vi "PH_AWG-510.set Status.vi"(0 "i ref in":refnum<vi>, 5 "error in":errorcluster) -> (14 "i ref out":refnum<vi>, 19 "error out":errorcluster)   [LabVIEW 2014, in "PH_AWG-510.lvlib"]
doc: "This VI sets the status: In case of a device failure it is set to failure (3), otherwise to on (2). The status is indicated and published a DIM-service."
uses:
  PH_AWG-510.lvlib
  PH_Basics/PH_StatusHandler/PH_StatusHandler.Status.ctl
  PH_Basics/PH_StatusHandler/PH_StatusHandler.lvlib
  instr.lib/awg510/Tektronix AWG510.lvlib
  PH_Basics/PH_Common/PH_Common.lvlib
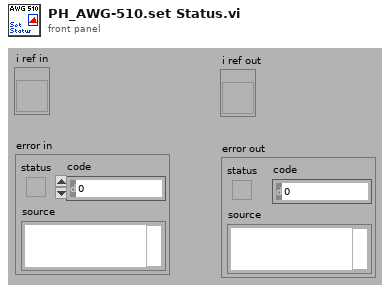
[diagram p1: front panel]
types:
  T1 = typedef "PH_AWG-510.lvlib/PH_AWG-510.i attribute.ctl" = cluster{"GUI Refs":cluster{"Delete":refnum<vi>, "Trigger Settings":refnum<vi>, "Start Device":refnum<vi>, "Instrument Information":refnum<vi>, "Lock Frontpanel":refnum<vi>, "Waveform Pattern File":refnum<vi>, "Initialize":refnum<vi>, "Output Settings":refnum<vi>}, "Instrument Information":T2, "Initialized?":bool, "Current Settings":cluster{"Trigger":T3, "Output Settings":T4}, "Wanted Settings":cluster{"Trigger":T3, "Output Settings":T4}, "Device frontpanel locked?":bool, "Default File Path":path}
  T2 = typedef "PH_AWG-510.lvlib/PH_AWG-510.Instrument Information Dataset.ctl" = cluster{"VISA resource name":refnum<visa-resource-name>, "Instrument Firmware Revision":string, "Manufacturer":string, "Model":string, "Serial Number":string, "Error Message":string, "Device Status":enum16{"stopped", "wating for trigger", "running", "Failure"}}
  T3 = typedef "PH_AWG-510.lvlib/PH_AWG-510.Trigger Settings.ctl" = cluster{"Mode":enum16{"Continuous", "Triggered", "Gated", "Enhanced"}, "Level (V)":dbl, "External Source":bool}
  T4 = typedef "PH_AWG-510.lvlib/PH_AWG-510.Output Settings.ctl" = cluster{"Activate Channel":bool, "VPP (V)":dbl, "Clock (Hz)":dbl, "File Name (Device)":string, "#1":u16, "#2":u16, "#3":u16, "#4":u16, "#5":u16, "#6":u16, "#7":u16, "#8":u16, "#9":u16, "#10":u16, "#11":u16, "#12":u16, "#13":u16, "#14":u16, "#15":u16, "#16":u16, "#17":u16, "#18":u16, "#19":u16, "#20":u16, "Offset (V)":dbl}
  T5 = typedef "PH_StatusHandler.lvlib/PH_StatusHandler.Status.ctl" = i16
  T6 = enum16{"stopped", "wating for trigger", "running"}
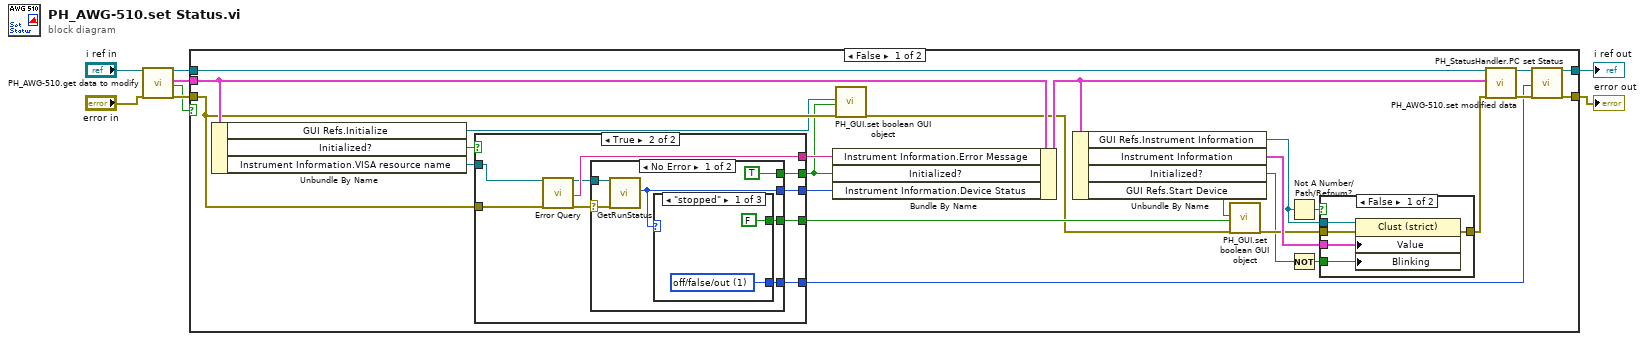
[diagram p0: block diagram]
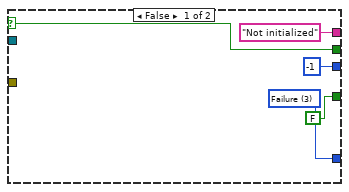
[diagram p2: hidden frame]
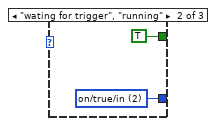
[diagram p3: hidden frame]
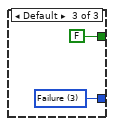
[diagram p4: hidden frame]
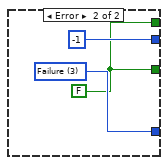
[diagram p5: hidden frame]
diagram:
  n1 = call "PH_AWG-510.get data to modify.vi"("i ref in"="i ref in", "error in (no error)"="error in") -> ("i ref out"=w7:refnum<vi>, "i attribute"=w3:T1, "timed out"=w1:bool, "error out"=w5:errorcluster)  [unwired: 14 in]
  n2 = case shown="False" w1 {
    tunnel: w7 -> [w33 w70]
    tunnel: w5 -> [w20 w69]
    tunnel: [w11 w70] -> w4
    tunnel: w3 -> [w32 _]
    tunnel: [w13 w69] -> w2
    frame False {
      n3 = Unbundle By Name(w32) -> ("GUI Refs.Initialize"=w14:refnum<vi>, "Initialized?"=w28:bool, "Instrument Information.VISA resource name"=w29:refnum<visa-resource-name>)
      n4 = case shown="True" w28 {
        selector: w28 -> [w36 _]
        tunnel: [w37 w47] -> w10
        tunnel: ["Not initialized" ("Error Message") w46] -> w17
        tunnel: w29 -> [_ w45]
        tunnel: w20 -> [_ w44]
        tunnel: [w36 w39] -> w15
        tunnel: [-1 w43] -> w24
        tunnel: [FALSE w42] -> w22
        frame False {
          w37 = T5 3 items=["no info", "off/false/out", "on/true/in", "Failure", "Alarm", "Status 1", "Status 2", "Status 3"] ("f")
        }
        frame True {
          n5 = call "Error Query.vi"("VISA resource name"=w45, "error in (no error)"=w44) -> ("VISA resource name out"=w41:refnum<visa-resource-name>, "Error Message"=w46:string, "error out"=w40:errorcluster)  [unwired: 14 in, 1 out]
          n6 = case shown="No Error" w40 {
            selector: w40 -> [w52 _]
            tunnel: w41 -> [w53 _]
            tunnel: [w51 -1] -> w43
            tunnel: [w50 w61] -> w47
            tunnel: [w49 w60] -> w42
            tunnel: [TRUE w60] -> w39
            frame No Error {
              n7 = call "GetRunStatus.vi"("VISA resource name"=w53, "error in"=w52) -> ("Status"=w51:T6)  [unwired: 15 in, 2 out]
              n8 = case shown="\"stopped\"" w51 {
                tunnel: [w55 w57 w59] -> w50
                tunnel: [FALSE TRUE FALSE] -> w49
                frame "stopped" {
                  w55 = T5 1 items=["no info", "off/false/out", "on/true/in", "Failure", "Alarm", "Status 1", "Status 2", "Status 3"] ("Status")
                }
                frame "wating for trigger", "running" {
                  w57 = T5 2 items=["no info", "off/false/out", "on/true/in", "Failure", "Alarm", "Status 1", "Status 2", "Status 3"] ("Status")
                }
                frame Default {
                  w59 = T5 3 items=["no info", "off/false/out", "on/true/in", "Failure", "Alarm", "Status 1", "Status 2", "Status 3"] ("Status")
                }
              }
            }
            frame Error {
              w60 = FALSE
              w61 = T5 3 items=["no info", "off/false/out", "on/true/in", "Failure", "Alarm", "Status 1", "Status 2", "Status 3"] ("Status")
            }
          }
        }
      }
      n9 = Bundle By Name(cluster=w32, "Instrument Information.Error Message"=w17, "Initialized?"=w15, "Instrument Information.Device Status"=w24) -> (w27:T1)
      n10 = call "PH_GUI.set boolean GUI object.vi"("Boolean Knob GUI Ref"=w14, "Value"=w15, "error in (no error)"=w20) -> ("error out"=w16:errorcluster)  [unwired: 16 in]
      n11 = Unbundle By Name(w27) -> ("GUI Refs.Instrument Information"=w25:refnum<vi>, "Instrument Information"=w26:T2, "Initialized?"=w19:bool, "GUI Refs.Start Device"=w21:refnum<vi>)
      n12 = call "PH_GUI.set boolean GUI object.vi"("Boolean Knob GUI Ref"=w21, "Value"=w22, "error in (no error)"=w16) -> ("error out"=w23:errorcluster)  [unwired: 16 in]
      n13 = Not A Number/Path/Refnum?(number/path/refnum=w25) -> (NaN/Path/Refnum?=w30:bool)
      n14 = Not(x=w19) -> (.not. x?=w18:bool)
      n15 = case shown="False" w30 {
        tunnel: w23 -> [w67 w68]
        tunnel: [w66 w68] -> w9
        tunnel: w25 -> [w65 _]
        tunnel: w18 -> [w63 _]
        tunnel: w26 -> [w64 _]
        frame False {
          n16 = property class="Clust (strict)"(reference=w65, error in=w67, "Value"=w64, "Blinking"=w63) -> (error out=w66:errorcluster)  [unwired: 1 out]
        }
        frame True {
        }
      }
      n17 = call "PH_AWG-510.set modified data.vi"("i ref in"=w33, "i attribute"=w27, "error in (no error)"=w9) -> ("i ref out"=w12:refnum<vi>, "error out"=w31:errorcluster)  [unwired: 15 in]
      n18 = call "PH_StatusHandler.PC set Status.vi"("i ref in"=w12, "Status"=w10, "error in (no error)"=w31) -> ("i ref out"=w11:refnum<vi>, "error out"=w13:errorcluster)  [unwired: 15 in]
    }
    frame True {
    }
  }
  "error out" <- w2
  "i ref out" <- w4
